vi "SingleAcquisition.vi"(8 "error in (no error)":errorcluster, 9 "Acq Number":u16, 10 "Image":T1, 11 "Hamamatsu_Camera in":refnum<class "Hamamatsu_Camera.lvclass">) -> (0 "error out":errorcluster, 3 "Hamamatsu_Camera out":refnum<class "Hamamatsu_Camera.lvclass">)   [LabVIEW 2023, in "Hamamatsu_Camera.lvlib" / "Hamamatsu_Camera.lvclass"]
uses:
  Hamamatsu_Camera.lvclass
  <vilib>/vision/Image Controls.llb/IMAQ Image.ctl
  <vilib>/ActorFramework/Actor/Actor.lvclass/Actor.ctl
  Hamamatsu_Camera.lvclass/Hamamatsu_Camera.ctl
  Interfaces/AbstractInstrumentClasses/Cameras_LV/CameraComm Messages/Frame Ready Msg/Frame Ready Msg.lvclass/Frame Ready Msg.ctl
  <vilib>/ActorFramework/Message Enqueuer/Message Enqueuer.lvclass/Message Enqueuer.ctl
  <vilib>/ActorFramework/Message Enqueuer/Enqueue.vi
  Interfaces/AbstractInstrumentClasses/Cameras_LV/CameraComm Messages/Frame Ready Msg/Frame Ready Msg.lvclass
  <vilib>/ActorFramework/Message Priority Queue/Priority Enqueue.vi
  <vilib>/ActorFramework/Actor/Actor.lvclass
  C:/Program Files/National Instruments/LabVIEW 2023/vi.lib/ActorFramework/Actor/Actor.lvclass
  C:/Users/quantum/Documents/LVDAQ/ConcreteClasses/ConcreteInstrumentClasses/CameraClasses/Hama_LV/HamaCam/Hamamatsu_Camera.lvclass
  C:/Users/quantum/Documents/LVDAQ/Interfaces/AbstractInstrumentClasses/Cameras_LV/CameraInterface/CameraInterface.lvclass
  C:/Users/quantum/Documents/LVDAQ/Interfaces/InitDeinitInterface/InitDeinit/InitDeinit.lvclass
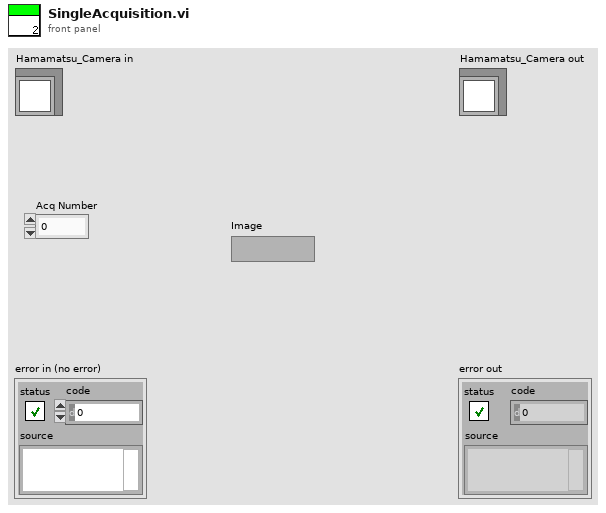
[diagram p1: front panel]
types:
  T1 = typedef "IMAQ Image.ctl" = refnum<image>
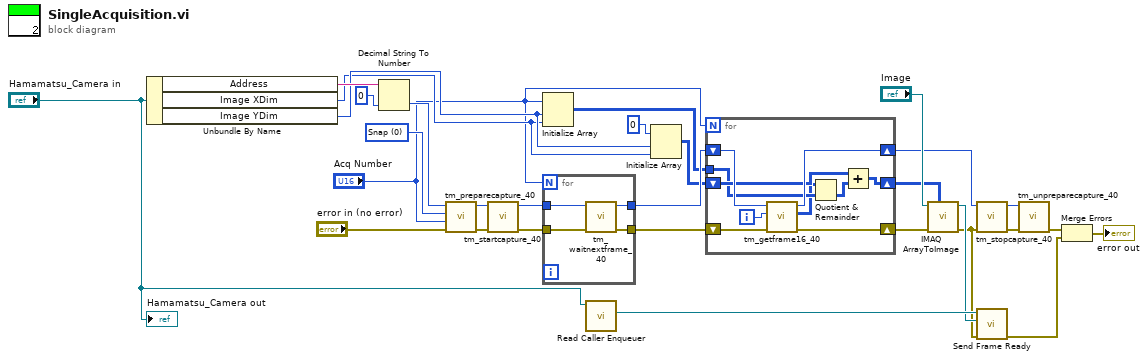
[diagram p0: block diagram]
diagram:
  w28 = 0 items=["Snap", "Sequence"] ("Capture mode")
  n1 = Unbundle By Name("Hamamatsu_Camera in") -> ("Address"=w21:string, "Image XDim"=w4:u16, "Image YDim"=w5:u16)
  n2 = Decimal String To Number(string=w21, default (0L)=u32 0 ("default (0 I32)")) -> (number=w23:u32)  [unwired: 1 in, 1 out]
  n3 = call "tm_preparecapture_40.vi"("error in (no error)"="error in (no error)", "Frames"="Acq Number", "Capture mode"=w28, "Handle in"=w23) -> ("error out"=w26:errorcluster, "Handle out"=w27:u32)  [unwired: 4 in, 2 out]
  n4 = call "tm_startcapture_40.vi"("error in (no error)"=w26, "Handle in"=w27) -> ("error out"=w13:errorcluster, "Handle out"=w12:u32)  [unwired: 8 in]
  n5 = Initialize Array("Acq Number", w5, w4) -> (w2:u16[][])
  n6 = for {
    N: "Acq Number" -> [_]
    tunnel: w13 -> [w34]
    tunnel: w12 -> [w33]
    tunnel: [w32] -> w11
    tunnel: [w31] -> w10
    n7 = call "tm_waitnextframe_40.vi"("error in (no error)"=w34, "Handle in"=w33) -> ("error out"=w32:errorcluster, "Handle out"=w31:u32)  [unwired: 6 in, 2 out]
  }
  n8 = call <vilib>:"Read Caller Enqueuer.vi"("Actor"="Hamamatsu_Camera in") -> ("Caller Enqueuer"=w20:refnum<class "Message Enqueuer.lvclass">)  [unwired: 10 in]
  n9 = Initialize Array(u8 0 ("element"), w5, w4) -> (w6:u8[][])
  n10 = for {
    N: "Acq Number" -> [_]
    shift-right: [w42] -> w9
    shift-left: w11 -> [w44]
    shift-right: [w41] -> w8
    shift-left: w10 -> [w43]
    shift-right: [w40] -> w1
    shift-left: w6 -> [w39]
    tunnel: w2 -> [w37]
    i -> [w38]
    n11 = call "tm_getframe16_40.vi"("error in (no error)"=w44, "Frame Index"=w38, "Handle in"=w43) -> ("error out"=w42:errorcluster, "Data"=w36:u16[][], "Handle out"=w41:u32)  [unwired: 5 in, 1 out]
    n12 = Quotient & Remainder(x=w36, y=w37) -> (floor(x/y)=w35:u16[][])  [unwired: 1 out]
    n13 = Add(x=w39, y=w35) -> (x+y=w40:u16[][])
  }
  n14 = call "IMAQ ArrayToImage"("Image Pixels (U16)"=w1, "error in (no error)"=w9, "Image"="Image") -> ("error out"=w17:errorcluster, "Image Out"=w18:T1)  [unwired: 7 in]
  n15 = call "tm_stopcapture_40.vi"("error in (no error)"=w17, "Handle in"=w8) -> ("error out"=w29:errorcluster, "Handle out"=w30:u32)  [unwired: 8 in]
  n16 = call "Send Frame Ready.vi"("error in (no error)"=w17, "Image In"=w18, "Message Enqueuer"=w20) -> ("error out"=w15:errorcluster)  [unwired: 7 in, 1 out]
  n17 = call "tm_unpreparecapture_40.vi"("error in (no error)"=w29, "Handle in"=w30) -> ("error out"=w16:errorcluster)  [unwired: 8 in, 1 out]
  n18 = Merge Errors(w16, w15) -> (→"error out":errorcluster)
  "Hamamatsu_Camera out" <- "Hamamatsu_Camera in"
